vi "Write VI Server Configuration.vi"(8 "error in (no error)":errorcluster, 10 "VI Server Configuration":T1, 11 "VI Server Recorder in":refnum<class "VI Server Recorder.lvclass">) -> (0 "error out":errorcluster, 3 "VI Server Recorder out":refnum<class "VI Server Recorder.lvclass">)   [LabVIEW 2019, in "VI Server Recorder.lvclass"]
uses:
  VI Server Recorder.lvclass
  C:/GitHub/LabActor/Template Module/Template Module.lvclass
  VI Server Configuration.ctl
  Template Module/Template Module.lvclass/Template Module.ctl
  Template Module/Write Configuration.vi
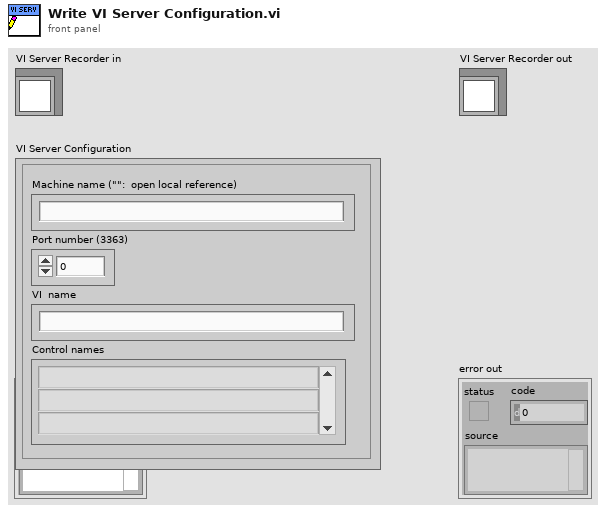
[diagram p1: front panel]
types:
  T1 = typedef "VI Server Configuration.ctl" = cluster{"Machine name (\"\":  open local reference)":string, "Port number (3363)":u16, "Control names":string[], "VI  name":string}
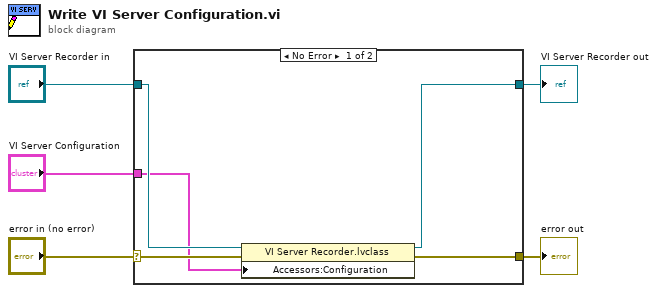
[diagram p0: block diagram]
diagram:
  n1 = case shown="No Error" "error in (no error)" {
    selector: "error in (no error)" -> [w10 w11]
    tunnel: [w9 w11] -> w4
    tunnel: [w7 w12] -> w2
    tunnel: "VI Server Recorder in" -> [w8 w12]
    tunnel: "VI Server Configuration" -> [w6 _]
    frame No Error {
      n2 = property class="VI Server Recorder.lvclass"(reference=w8, error in=w10, "Accessors:Configuration"=w6) -> (reference out=w7:refnum<class "VI Server Recorder.lvclass">, error out=w9:errorcluster)
    }
    frame Error {
    }
  }
  "error out" <- w4
  "VI Server Recorder out" <- w2
